vi "calcSummaryStiffnesses.vi"(8 "error in (no error)":errorcluster, 11 "StiffnessCalculator in":refnum<class "StiffnessCalculator.lvclass">) -> (0 "error out":errorcluster, 3 "StiffnessCalculator out":refnum<class "StiffnessCalculator.lvclass">)   [LabVIEW 2015, in "StiffnessCalculator.lvclass"]
uses:
  StiffnessCalculator.lvclass
  StiffnessCalculator.lvclass/StiffnessCalculator.ctl
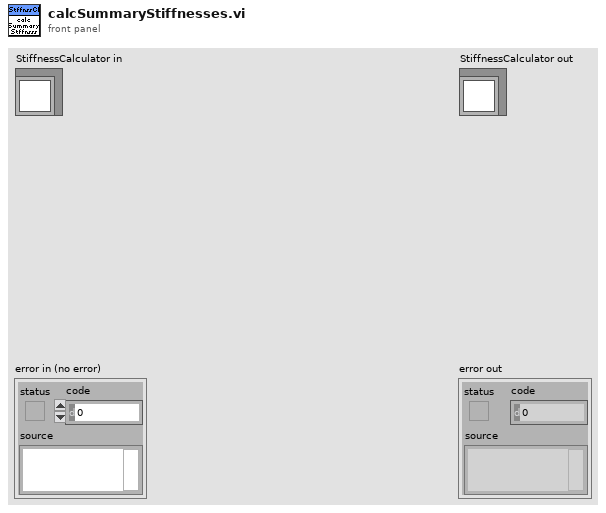
[diagram p1: front panel]
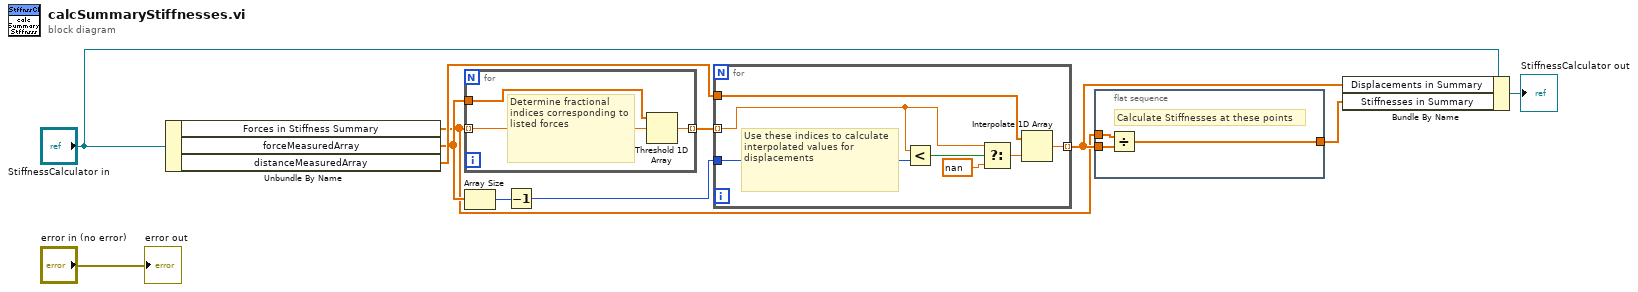
[diagram p0: block diagram]
diagram:
  n1 = Unbundle By Name("StiffnessCalculator in") -> ("Forces in Stiffness Summary"=w3:dbl[unit][], "forceMeasuredArray"=w5:dbl[unit][], "distanceMeasuredArray"=w9:dbl[unit][])
  n2 = for {
    tunnel: w5 -> [w14]
    tunnel: w3 -> [w13] mode=indexing
    tunnel: [w12] -> w2 mode=indexing
    # "Determine fractional indices corresponding to listed forces"
    n3 = Threshold 1D Array(2:w13, 3:w14) -> (0:w12:dbl)  [unwired: 1 in]
  }
  n4 = Array Size(array=w5) -> (size(s)=w4:i32)
  n5 = Decrement(x=w4) -> (x-1=w1:i32)
  n6 = for {
    tunnel: w2 -> [w17] mode=indexing
    tunnel: w9 -> [w21]
    tunnel: [w20] -> w8 mode=indexing
    tunnel: w1 -> [w19]
    # "Use these indices to calculate interpolated values for displacements"
    n7 = Less?(x=w17, y=w19) -> (x < y?=w18:bool)
    n8 = Select(t=w17, s=w18, f=nan) -> (s? t:f=w16:dbl)
    n9 = Interpolate 1D Array(1:w16, 2:w21) -> (0:w20:dbl[unit])
  }
  n10 = flat-sequence {
    tunnel: w3 -> [w24]
    tunnel: w8 -> [w23]
    tunnel: [w22] -> w7
    frame #0 {
      # "Calculate Stiffnesses at these points"
      n11 = Divide(x=w24, y=w23) -> (x/y=w22:dbl[unit][])
    }
  }
  n12 = Bundle By Name(cluster="StiffnessCalculator in", "Displacements in Summary"=w8, "Stiffnesses in Summary"=w7) -> (→"StiffnessCalculator out":refnum<class "StiffnessCalculator.lvclass">)
  "error out" <- "error in (no error)"
